vi "portada_reporte_subvi.vi"(8 "Final":timestamp, 9 "Inicio":timestamp, 10 "Numeric":i32, 11 "Numeric 2":i32) -> ()   [LabVIEW 2021]
uses:
  <vilib>/Utility/NIReport.llb/Report Type.ctl
  <vilib>/Utility/NIReport.llb/Append Report Text (str wrap).vi
  <vilib>/Utility/NIReport.llb/NI_report.lvclass
  <vilib>/Utility/NIReport.llb/NI_ReportGenerationCore.lvlib
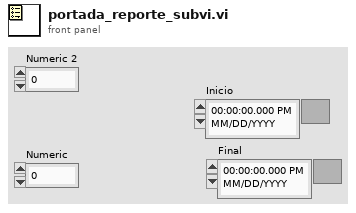
[diagram p1: front panel]
types:
  T1 = cluster{"Charset (-1)":i16, "Weight (-1)":i16, "Name":string, "Size":string}
  T2 = cluster{"Italic":enum16{"Italic Unchanged", "Italic On", "Italic Off"}, "Strike Through":enum16{"Strike Through Unchanged", "Strike Through On", "Strike Through Off"}, "Underline":enum16{"Underline Unchanged", "Underline On", "Underline Off"}, "Bold":enum16{"Bold Unchanged", "Bold On", "Bold Off"}}
  T3 = typedef "NI_ReportGenerationCore.lvlib/Report Type.ctl" = enum16{"HTML", "Word", "Excel"}
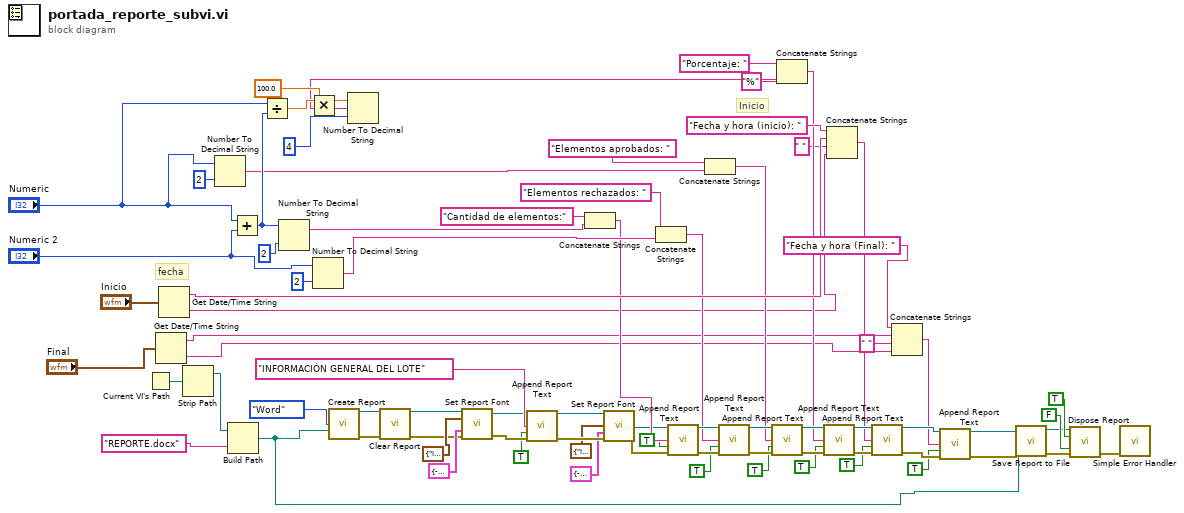
[diagram p0: block diagram]
diagram:
  # "Inicio"
  # "fecha"
  n1 = Current VI's Path() -> (path=w23:path)
  n2 = Get Date/Time String(seconds (now)="Final") -> (date string=w14:string, time string=w6:string)  [unwired: 2 in]
  n3 = Get Date/Time String(seconds (now)="Inicio") -> (date string=w64:string, time string=w8:string)  [unwired: 2 in]
  n4 = Strip Path(path=w23) -> (stripped path=w25:path)  [unwired: 1 out]
  n5 = Number To Decimal String(number="Numeric", width (-)=i16 2) -> (decimal integer string=w54:string)
  n6 = Build Path(base path=w25, name or relative path="REPORTE.docx") -> (appended path=w79:path)
  n7 = Add(x="Numeric", y="Numeric 2") -> (x+y=w57:i32)
  n8 = Divide(x="Numeric", y=w57) -> (x/y=w59:dbl)
  n9 = Number To Decimal String(number=w57, width (-)=i16 2) -> (decimal integer string=w47:string)
  n10 = Multiply(x=w59, y=100.0) -> (x*y=w12:dbl)
  n11 = Number To Decimal String(number="Numeric 2", width (-)=i16 2) -> (decimal integer string=w50:string)
  n12 = call <vilib>:"Create Report.vi"("report type"=Report_Type."Word", "template (empty)"=w79) -> ("report out"=w4:refnum<class "NI_report.lvclass">, "error out"=w3:errorcluster)  [unwired: 12 in]
  n13 = Number To Decimal String(number=w12, width (-)=i16 4) -> (decimal integer string=w10:string)
  n14 = call-dynamic "Clear Report.vi"("report in"=w4, "error in (no error)"=w3) -> ("report out"=w2:refnum<class "NI_report.lvclass">, "error out"=w1:errorcluster)  [unwired: 12 in]
  n15 = call-dynamic "Set Report Font.vi"("report in"=w2, "text options"=T2 {"Italic"=enum."Italic Unchanged", "Strike Through"=enum."Strike Through Unchanged", "Underline"=enum."Underline Unchanged", "Bold"=enum."Bold On"}, "font settings"=T1 {"Charset (-1)"=-1, "Weight (-1)"=-1, "Name"="Arial", "Size"="18 "}, "error in (no error)"=w1) -> ("report out"=w31:refnum<class "NI_report.lvclass">, "error out"=w32:errorcluster)  [unwired: 9 in, 1 out]
  n16 = call-poly <vilib>:"Append Report Text.vi"("report in"=w31, "text"="INFORMACIÓN GENERAL DEL LOTE", "append on new line? (F)"=TRUE, "error in (no error)"=w32) -> ("report out"=w36:refnum<class "NI_report.lvclass">, "error out"=w37:errorcluster)  [unwired: 8 in, 2 out]
  n17 = Concatenate Strings("Cantidad de elementos:" ("text"), w47) -> (w45:string)
  n18 = call-dynamic "Set Report Font.vi"("report in"=w36, "text options"=T2 {"Italic"=enum."Italic Unchanged", "Strike Through"=enum."Strike Through Unchanged", "Underline"=enum."Underline Unchanged", "Bold"=enum."Bold On"}, "font settings"=T1 {"Charset (-1)"=-1, "Weight (-1)"=-1, "Name"="Arial", "Size"="17 "}, "error in (no error)"=w37) -> ("report out"=w38:refnum<class "NI_report.lvclass">, "error out"=w39:errorcluster)  [unwired: 9 in, 1 out]
  n19 = Concatenate Strings("Elementos rechazados: " ("text"), w50) -> (w52:string)
  n20 = call-poly <vilib>:"Append Report Text.vi"("report in"=w38, "text"=w45, "append on new line? (F)"=TRUE, "error in (no error)"=w39) -> ("report out"=w70:refnum<class "NI_report.lvclass">, "error out"=w71:errorcluster)  [unwired: 8 in, 2 out]
  n21 = Concatenate Strings("Elementos aprobados: " ("text"), w54) -> (w56:string)
  n22 = call-poly <vilib>:"Append Report Text.vi"("report in"=w70, "text"=w52, "append on new line? (F)"=TRUE, "error in (no error)"=w71) -> ("report out"=w69:refnum<class "NI_report.lvclass">, "error out"=w72:errorcluster)  [unwired: 8 in, 2 out]
  n23 = call-poly <vilib>:"Append Report Text.vi"("report in"=w69, "text"=w56, "append on new line? (F)"=TRUE, "error in (no error)"=w72) -> ("report out"=w68:refnum<class "NI_report.lvclass">, "error out"=w73:errorcluster)  [unwired: 8 in, 2 out]
  n24 = Concatenate Strings("Porcentaje: " ("text"), w10, "%" ("string")) -> (w62:string)
  n25 = call-poly <vilib>:"Append Report Text.vi"("report in"=w68, "text"=w62, "append on new line? (F)"=TRUE, "error in (no error)"=w73) -> ("report out"=w66:refnum<class "NI_report.lvclass">, "error out"=w67:errorcluster)  [unwired: 8 in, 2 out]
  n26 = Concatenate Strings("Fecha y hora (inicio): " ("text"), w64, " " ("string"), w8) -> (w65:string)
  n27 = call-poly <vilib>:"Append Report Text.vi"("report in"=w66, "text"=w65, "append on new line? (F)"=TRUE, "error in (no error)"=w67) -> ("report out"=w21:refnum<class "NI_report.lvclass">, "error out"=w19:errorcluster)  [unwired: 8 in, 2 out]
  n28 = Concatenate Strings("Fecha y hora (Final): " ("text"), w14, " " ("string"), w6) -> (w16:string)
  n29 = call-poly <vilib>:"Append Report Text.vi"("report in"=w21, "text"=w16, "append on new line? (F)"=TRUE, "error in (no error)"=w19) -> ("report out"=w20:refnum<class "NI_report.lvclass">, "error out"=w18:errorcluster)  [unwired: 8 in, 2 out]
  n30 = call-dynamic "Save Report to File.vi"("report in"=w20, "report file path"=w79, "error in (no error)"=w18) -> ("report out"=w74:refnum<class "NI_report.lvclass">, "error out"=w75:errorcluster)  [unwired: 11 in]
  n31 = call-dynamic "Dispose Report.vi"("report in"=w74, "wait until printing completed? (T)"=TRUE, "save changes? (F)"=FALSE, "error in (no error)"=w75) -> ("error out"=w76:errorcluster)  [unwired: 11 in]
  n32 = call <vilib>:"Simple Error Handler.vi"("error in (no error)"=w76) -> ()  [unwired: 4 in, 5 out]
